vi "Group ID to Tree Items.vi"(8 "error in (no error)":errorcluster, 9 "Group ID":string, 10 "Indent":i32, 11 "Application Data in":T1) -> (0 "error out":errorcluster, 2 "Items":T3(array[cluster]), 3 "Application Data out":T1)   [LabVIEW 2017]
uses:
  Application Data.ctl
  DSF Configuration API/1.0.0/Public/Controls/DSF Config Data RefNum.ctl
  Window State.ctl
  Tree Item Type.ctl
  DSF Configuration API/1.0.0/Public/Read Item/Read Group.vi
  DSF Configuration API/1.0.0/Public/Read Item/Read Settings.vi
  DSF Configuration API/1.0.0/DSF Configuration API.lvlib
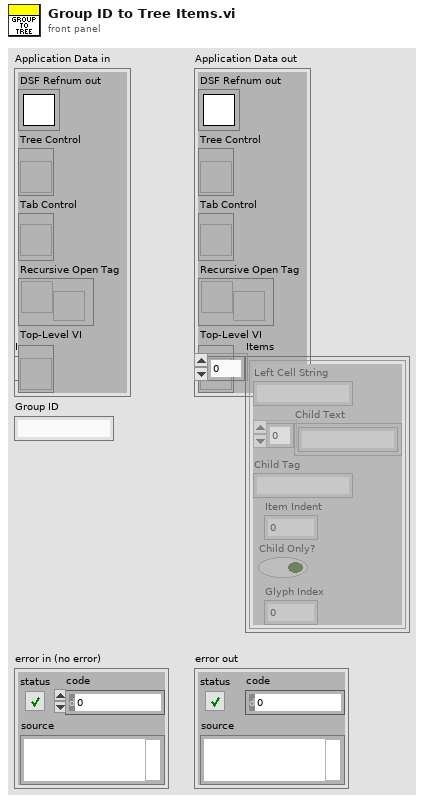
[diagram p1: front panel]
types:
  T1 = typedef "Application Data.ctl" = cluster{"DSF Refnum out":T2, "Tree Control":refnum<vi>, "Tab Control":refnum<vi>, "Recursive Open Tag":refnum<user-event>, "Top-Level VI":refnum<vi>}
  T2 = typedef "DSF Configuration API.lvlib/DSF Config Data RefNum.ctl" = refnum<k1>
  T3 = cluster{"Left Cell String":string, "Child Text":string[], "Child Tag":string, "Item Indent":i32, "Child Only?":bool, "Glyph Index":i32}[]
  T4 = typedef "Tree Item Type.ctl" = enum16{"Plugin", "Group", "Transfer", "Channel", "Setting"}
  T5 = typedef "DSF Configuration API.lvlib/DSF Group Info.ctl" = cluster{"direction":i32, "timing":T6, "transfer ids":string[], "settings id":string}
  T6 = typedef "DSF Configuration API.lvlib/DSF Timing Info.ctl" = cluster{"decimation":i32, "offset":i32}
  T7 = cluster{"Left Cell String":string, "Child Text":string[], "Child Tag":string, "Item Indent":i32, "Child Only?":bool, "Glyph Index":i32}
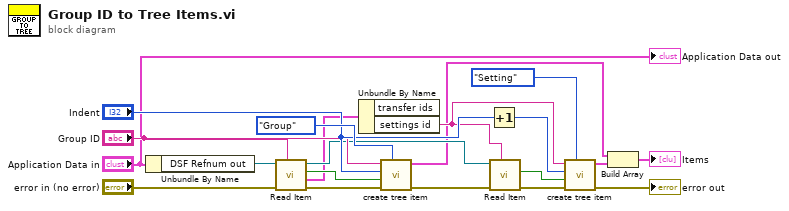
[diagram p0: block diagram]
diagram:
  n1 = Unbundle By Name("Application Data in") -> ("DSF Refnum out"=w1:T2)
  n2 = call-poly "Read Item.vi"("name"="Group ID", "error in (no error)"="error in (no error)", "refnum"=w1) -> ("error out"=w16:errorcluster, "value"=w7:T5, "found?"=w13:bool, "refnum out"=w9:T2)  [unwired: 5 in]
  n3 = Unbundle By Name(w7) -> ("settings id"=w11:string)  [unwired: 1 out]
  n4 = call "create tree item.vi"("Item Type"=Tree_Item_Type."Group", "error in"=w16, "found?"=w13, "Indent"="Indent", "Left Cell String"="Group ID") -> ("error out"=w17:errorcluster, "Item"=w5:T7)  [unwired: 5 in]
  n5 = Increment(x="Indent") -> (x+1=w15:i32)
  n6 = call-poly "Read Item.vi"("name"=w11, "error in (no error)"=w17, "refnum"=w9) -> ("error out"=w18:errorcluster, "found?"=w14:bool)  [unwired: 5 in, 2 out]
  n7 = call "create tree item.vi"("Item Type"=Tree_Item_Type."Setting", "error in"=w18, "found?"=w14, "Indent"=w15, "Left Cell String"=w11) -> ("error out"=→"error out":errorcluster, "Item"=w4:T7)  [unwired: 5 in]
  n8 = Build Array(w5, w4) -> (→"Items":T3)
  "Application Data out" <- "Application Data in"
